vi "svc_Get SV Channel Info.vi"(6 "channel index":i32, 8 "error in (no error)":errorcluster, 11 "scaled signal [EU]":waveform(dbl)={"t0"=timestamp(0 s since 1904-01-01), "dt"=0.0, "Y"=[]}) -> (0 "error out":errorcluster, 1 "unit label":string, 2 "channel info":T1={"sensor sensitivity"=1000.0, "engineering units"=1, "dB reference"=1.0, "custom label"="EU", "weighting filter"=0, "pregain"=0.0} {"pregain" format="%.2f"; "weighting filter" items=["Linear", "A-weighting", "B-weighting", "C-weighting", "ITU-R 468-4", "Dolby", "CCITT", "C-message", "Wb", "Wc", "Wd", "We", "Wf", "Wh", "Wj", "Wk", "Wm", "AES17 20 kHz lowpass", "AES17 40 kHz lowpass", "AES17 20 kHz highpass", "AES17 40 kHz highpass"]; "dB reference" format="%^.1e"; "engineering units" items=["custom..."=0, "V"=1, "A"=21, "C"=30, "pC"=31, "s"=32, "-"=29, "Pa"=2, "N"=20, "g"=3, "m/s^2"=4, "m/s"=5, "m"=6, "mm/s"=12, "mm"=13, "micron/s"=14, "micron"=15, "in/s^2"=7, "in/s"=8, "in"=9, "mil/s"=10, "mil"=11, "rad/s^2"=16, "rad/s"=17, "rad"=18, "deg/s^2"=26, "deg/s"=27, "deg"=28, "RPM"=22, "cycle/s^2"=23, "Hz"=24, "cycle"=25, "strain"=19]; "sensor sensitivity" format="%#_5f"}, 3 "dup scaled signal [EU]":waveform(dbl), 5 "channel name":string, 7 "channel description":string)   [LabVIEW 2017]
uses:
  <vilib>/addons/_NISVFA/_Shared subVIs/Controls/svc_Channel Info.ctl
  <vilib>/addons/_NISVFA/_Shared subVIs/Controls/svc_Engineering Units Text Ring.ctl
  <vilib>/addons/_NISVFA/_Shared subVIs/Controls/svc_Weighting Filter Text Ring.ctl
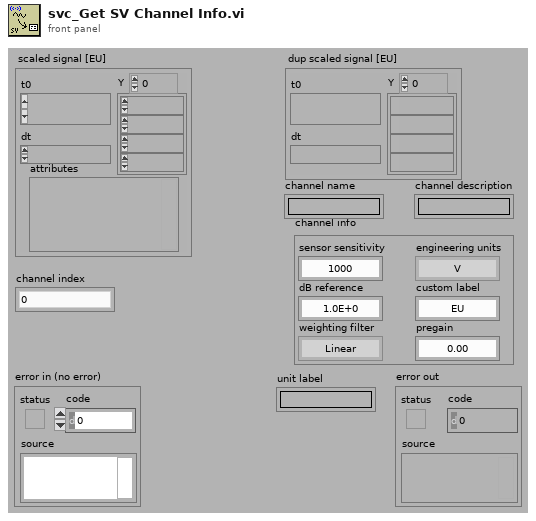
[diagram p1: front panel]
types:
  T1 = typedef "svc_Channel Info.ctl" = cluster{"sensor sensitivity":dbl, "engineering units":T2, "dB reference":dbl, "custom label":string, "weighting filter":T3, "pregain":dbl}
  T2 = typedef "svc_Engineering Units Text Ring.ctl" = u16
  T3 = typedef "svc_Weighting Filter Text Ring.ctl" = u16
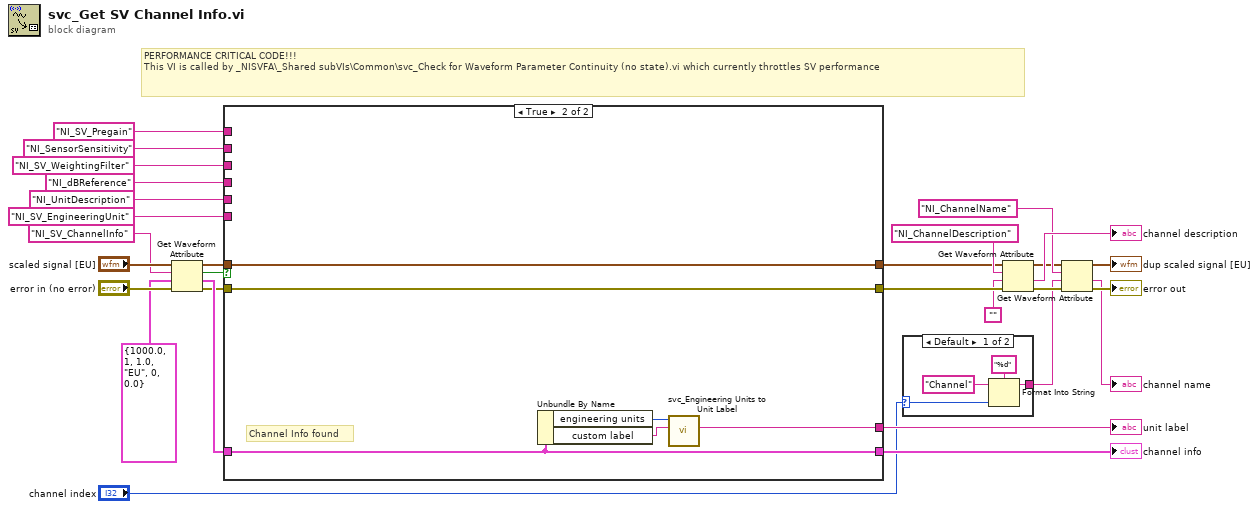
[diagram p0: block diagram]
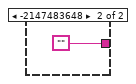
[diagram p2: hidden frame]
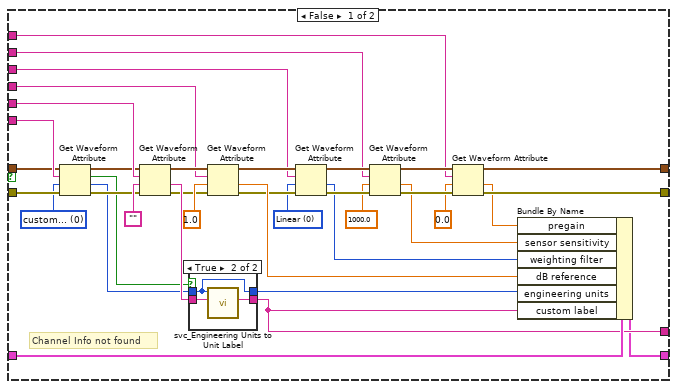
[diagram p3: hidden frame]
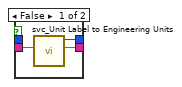
[diagram p4: hidden frame]
diagram:
  # "PERFORMANCE CRITICAL CODE!!!\nThis VI is called by _NISVFA\\_Shared subVIs\\Common\\svc_Check for Waveform Parameter Continuity (no state).vi which currently throttles SV performance"
  n1 = Get Waveform Attribute(4:"error in (no error)", 5:T1 {"sensor sensitivity"=1000.0, "engineering units"=1, "dB reference"=1.0, "custom label"="EU", "weighting filter"=0, "pregain"=0.0} ("channel info"), 6:"NI_SV_ChannelInfo" ("name"), 7:"scaled signal [EU]") -> (0:w17:errorcluster, 1:w18:T1, 2:w20:bool, 3:w19:waveform(dbl))
  n2 = case shown="True" w20 {
    tunnel: w19 -> [w54 w77]
    tunnel: [w30 w76] -> w28
    tunnel: w18 -> [w63 w76]
    tunnel: w17 -> [w55 w78]
    tunnel: [w36 w78] -> w11
    tunnel: [w35 w77] -> w14
    tunnel: [w31 w73] -> w22
    tunnel: "NI_dBReference" ("name") -> [w58 _]
    tunnel: "NI_UnitDescription" ("name") -> [w57 _]
    tunnel: "NI_SV_EngineeringUnit" ("name") -> [w56 _]
    tunnel: "NI_SV_WeightingFilter" ("name") -> [w42 _]
    tunnel: "NI_SensorSensitivity" ("name") -> [w41 _]
    tunnel: "NI_SV_Pregain" ("name") -> [w40 _]
    frame False {
      w39 = T3 0 items=["Linear", "A-weighting", "B-weighting", "C-weighting", "ITU-R 468-4", "Dolby", "CCITT", "C-message"] ("weighting filter")
      w51 = T2 0 items=["custom..."=0, "V"=1, "A"=21, "Pa"=2, "N"=20, "g"=3, "m/s^2"=4, "m/s"=5, "m"=6, "mm/s"=12, "mm"=13, "micron/s"=14, "micron"=15, "in/s^2"=7, "in/s"=8, "in"=9, "mil/s"=10, "mil"=11, "rad/s^2"=16, "rad/s"=17, "rad"=18, "strain"=19] ("engineering units")
      # "Channel Info not found"
      n3 = Get Waveform Attribute(4:w55, 5:w51, 6:w56, 7:w54) -> (0:w52:errorcluster, 1:w49:T2, 2:w50:bool, 3:w53:waveform(dbl))
      n4 = Get Waveform Attribute(4:w52, 5:"" ("Empty String Constant"), 6:w57, 7:w53) -> (0:w59:errorcluster, 1:w65:string, 3:w60:waveform(dbl))  [unwired: 1 out]
      n5 = case shown="True" w50 {
        tunnel: w65 -> [w69 w71]
        tunnel: [w68 w70] -> w64
        tunnel: [w67 w72] -> w31
        tunnel: w49 -> [_ w70]
        frame False {
          n6 = call <vilib>:"svc_Unit Label to Engineering Units.vi"("unit label"=w69) -> ("unit label out"=w67:string, "engineering units"=w68:T2)  [unwired: 9 in]
        }
        frame True {
          n7 = call <vilib>:"svc_Engineering Units to Unit Label.vi"("custom label"=w71, "engineering units"=w70) -> ("unit label"=w72:string)  [unwired: 8 in, 1 out]
        }
      }
      n8 = Get Waveform Attribute(4:w59, 5:1.0, 6:w58, 7:w60) -> (0:w47:errorcluster, 1:w61:dbl, 3:w48:waveform(dbl))  [unwired: 1 out]
      n9 = Get Waveform Attribute(4:w47, 5:w39, 6:w42, 7:w48) -> (0:w46:errorcluster, 1:w33:T3, 3:w45:waveform(dbl))  [unwired: 1 out]
      n10 = Get Waveform Attribute(4:w46, 5:1000.0 ("sensor sensitivity [mV/EU]"), 6:w41, 7:w45) -> (0:w44:errorcluster, 1:w34:dbl, 3:w43:waveform(dbl))  [unwired: 1 out]
      n11 = Get Waveform Attribute(4:w44, 5:0.0 ("pregain [dB]"), 6:w40, 7:w43) -> (0:w36:errorcluster, 1:w32:dbl, 3:w35:waveform(dbl))  [unwired: 1 out]
      n12 = Bundle By Name(cluster=w63, "pregain"=w32, "sensor sensitivity"=w34, "weighting filter"=w33, "dB reference"=w61, "engineering units"=w64, "custom label"=w31) -> (w30:T1)
    }
    frame True {
      # "Channel Info found"
      n13 = Unbundle By Name(w76) -> ("engineering units"=w75:T2, "custom label"=w74:string)
      n14 = call <vilib>:"svc_Engineering Units to Unit Label.vi"("custom label"=w74, "engineering units"=w75) -> ("unit label"=w73:string)  [unwired: 8 in, 1 out]
    }
  }
  "channel info" <- w28
  "unit label" <- w22
  n15 = case shown="Default" "channel index" {
    selector: "channel index" -> [w80 _]
    tunnel: [w79 "" ("Empty String Constant")] -> w2
    frame Default {
      n16 = Format Into String(format string="%d", initial string="Channel" ("string"), w80) -> (resulting string=w79:string)  [unwired: 1 in, 1 out]
    }
    frame -2147483648 {
    }
  }
  n17 = Get Waveform Attribute(4:w11, 5:"" ("Empty String Constant"), 6:"NI_ChannelDescription" ("name"), 7:w14) -> (0:w12:errorcluster, 1:→"channel description":string, 3:w13:waveform(dbl))  [unwired: 1 out]
  n18 = Get Waveform Attribute(4:w12, 5:w2, 6:"NI_ChannelName" ("name"), 7:w13) -> (0:→"error out":errorcluster, 1:→"channel name":string, 3:→"dup scaled signal [EU]":waveform(dbl))  [unwired: 1 out]
